vi "Send Single Message To Specific Target.vi"(6 "Paras In":variant, 7 "Priority":i32, 8 "error in (no error)":errorcluster, 9 "Mail Strategy In":refnum<class "Mail Strategy.lvclass">, 10 "Message In":refnum<class "Message.lvclass">, 11 "Simple Map Queue Group Messenger in":refnum<class "Simple Map Queue Group Messenger.lvclass">) -> (0 "error out":errorcluster, 3 "Simple Map Queue Group Messenger out":refnum<class "Simple Map Queue Group Messenger.lvclass">)   [LabVIEW 2024, in "Simple Map Queue Group Messenger.lvclass"]
uses:
  Simple Map Queue Group Messenger.lvclass
  Ancestor Class/Message/Message.lvclass
  Ancestor Class/Messenger/Mail Strategy/Mail Strategy.lvclass
  Simple Map Queue Group Messenger.lvclass/Simple Map Queue Group Messenger.ctl
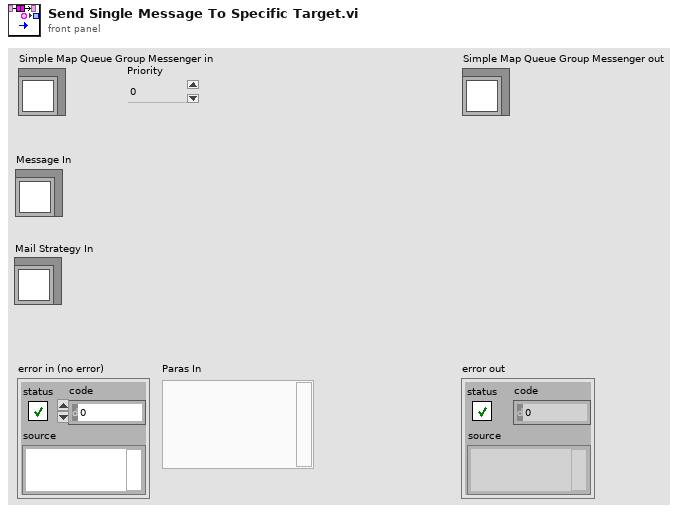
[diagram p1: front panel]
types:
  T1 = typedef "Queue Group Map.ctl" = map{i64, T2[]}
  T2 = typedef "Message Queue.ctl" = refnum<queue>
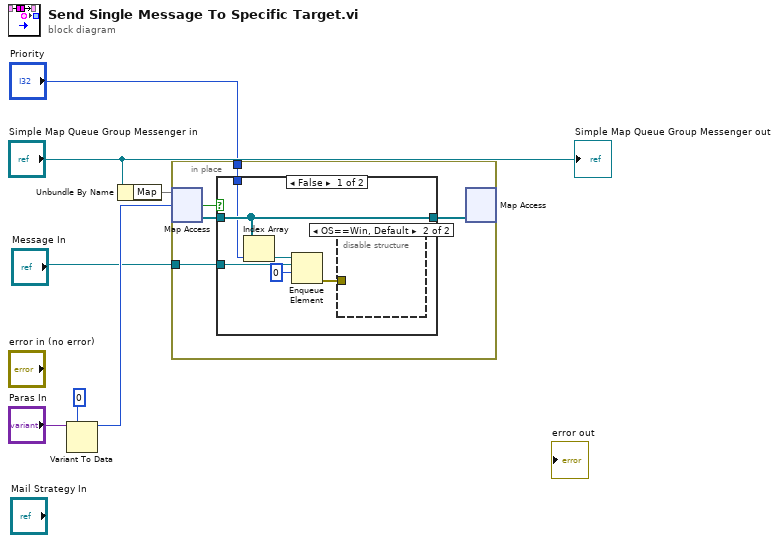
[diagram p0: block diagram]
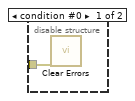
[diagram p2: hidden frame]
diagram:
  n1 = Variant To Data(type=i64 0, Variant="Paras In") -> (data=w5:i64)  [unwired: 1 in, 1 out]
  n2 = Unbundle By Name("Simple Map Queue Group Messenger in") -> ("Map"=w7:T1)
  n3 = in-place {
    in-place-border: "Message In" -> [w9]
    in-place-border: "Priority" -> [w8]
    n4 = in-place-map #1(w7, w5) -> (w11:T2[], w12:bool)  [unwired: 1 in]
    n5 = case shown="False" w12 {
      tunnel: w11 -> [w17 w20]
      tunnel: [w17 w20] -> w10
      tunnel: w9 -> [w16 _]
      tunnel: w8 -> [w15 _]
      frame False {
        n6 = Index Array(array=w17, index=w15) -> (element=w18:T2)
        n7 = Enqueue Element(queue=w18, element=w16, timeout in ms (-1)=0) -> (error out=w13:errorcluster)  [unwired: 1 in, 2 out]
        n8 = disable-structure shown="OS==Win, Default" {
          disable-tunnel: w13 -> [w19 _]
          frame condition #0 {
            n9 = call <vilib>:"Clear Errors.vi"("error in (no error)"=w19) -> ()  [unwired: 5 in, 2 out]
          }
          frame condition #1 (active) {
          }
        }
      }
      frame True {
      }
    }
    n10 = in-place-map #1(w10) -> ()  [unwired: 1 in, 3 out]
  }
  "Simple Map Queue Group Messenger out" <- "Simple Map Queue Group Messenger in"
